vi "Prompt for Step.vi"(8 "error in (no error)":errorcluster, 9 "Exit Event":refnum<user-event>, 10 "Subpanel Ref":refnum<vi>, 11 "Keyboard Action in":refnum<class "Keyboard Action.lvclass">) -> (0 "error out":errorcluster, 2 "OK?":bool, 3 "Keyboard Action out":refnum<class "Keyboard Action.lvclass">)   [LabVIEW 2020, in "MacroAssert.lvlib" / "Keyboard Action.lvclass"]
uses:
  Keyboard Action.lvclass
  Keyboard Action.lvclass/Keyboard Action.ctl
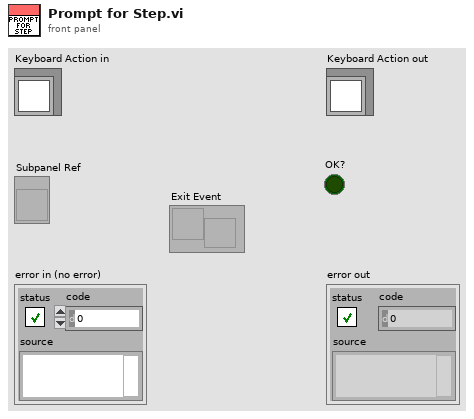
[diagram p1: front panel]
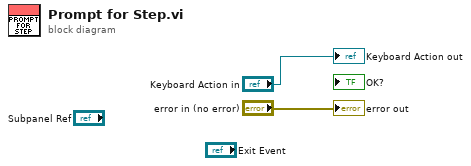
[diagram p0: block diagram]
diagram:
  "error out" <- "error in (no error)"
  "Keyboard Action out" <- "Keyboard Action in"
